vi "Practice_MultipleVariableStringOutput.vi"() -> ()   [LabVIEW 2014]
panel:
  out "String":string
  in  "stop":bool
  in  "Update":bool
  in  "I dont even know":dbl
  in  "Weenie Hut Jr.":dbl
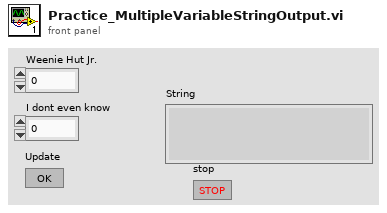
[diagram p1: front panel]
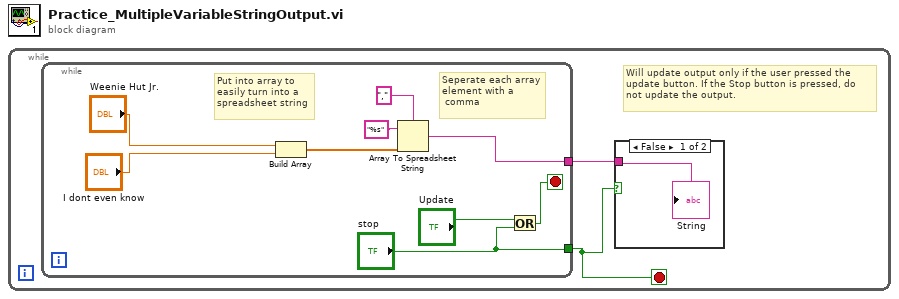
[diagram p0: block diagram]
diagram:
  n1 = while {
    stop <- w1 stop-if-true
    # "Will update output only if the user pressed the \nupdate button. If the Stop button is pressed, do\nnot update the output."
    n2 = while {
      tunnel: ["stop"] -> w1
      tunnel: [w4] -> w2
      stop <- w7 stop-if-true
      # "Seperate each array\nelement with a\n comma"
      # "Put into array to \neasily turn into a \nspreadsheet string"
      n3 = Build Array("Weenie Hut Jr.", "I dont even know") -> (w10:dbl[])
      n4 = Array To Spreadsheet String(delimiter (Tab)=",", array=w10, 3:"%s" ("format string")) -> (spreadsheet string=w4:string)
      n5 = Or(x="Update", y="stop") -> (x .or. y?=w7:bool)
    }
    n6 = case shown="False" w1 {
      tunnel: w2 -> [w3 _]
      frame False {
        "String" <- w3
      }
      frame True {
      }
    }
  }
